vi "Auto Dispose.vi"(8 "error in (no error)":errorcluster, 11 "Progress Bar":refnum<data-value>) -> (0 "error out":errorcluster, 3 "Progress Bar":refnum<data-value>)   [LabVIEW 2016, in "Progress Bar.lvclass"]
doc: "If the reference was auto generated, then this VI will dispose of it when the progress bar is complete\n\nCopyright: MGI\nAuthored by: Derek Trepanier"
uses:
  <userlib>/_MGI/User Interface/Progress Bar/Progress Bar.lvclass
  <userlib>/_MGI/User Interface/Progress Bar/Progress Bar.lvclass/Progress Bar.ctl
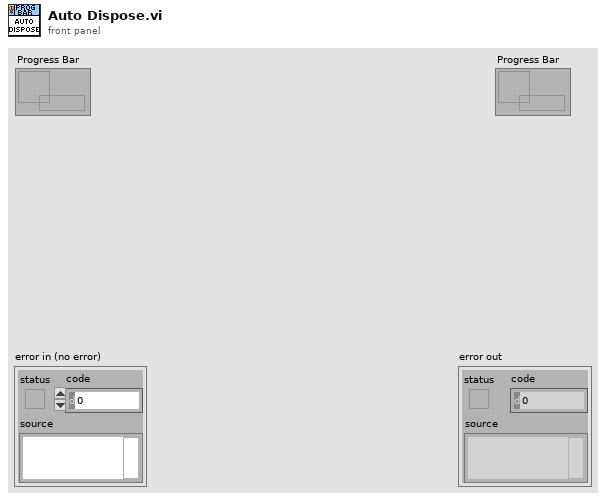
[diagram p1: front panel]
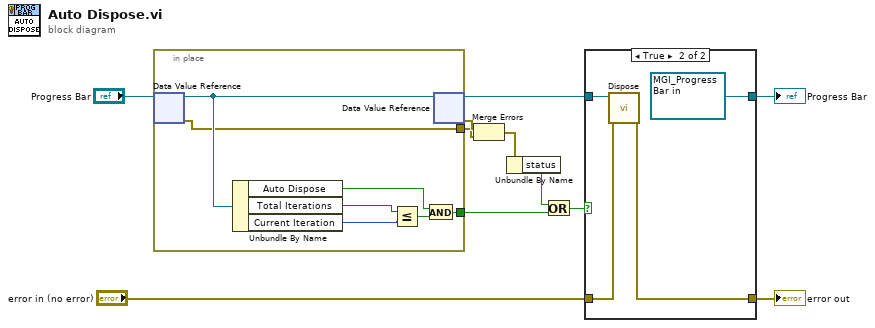
[diagram p0: block diagram]
diagram:
  n1 = in-place {
    in-place-border: [w14] -> w6
    in-place-border: [w13] -> w1
    n2 = in-place-dvr #1("Progress Bar") -> (w18:refnum<class "Progress Bar.lvclass">, w13:errorcluster)
    n3 = Unbundle By Name(w18) -> ("Auto Dispose"=w15:bool, "Total Iterations"=w17:i32, "Current Iteration"=w12:i32)
    n4 = Less Or Equal?(x=w17, y=w12) -> (x <= y?=w16:bool)
    n5 = And(x=w15, y=w16) -> (x .and. y?=w14:bool)
    n6 = in-place-dvr #1(w18) -> (w7:refnum<data-value>, w2:errorcluster)
  }
  n7 = Merge Errors(w2, w1) -> (w4:errorcluster)
  n8 = Unbundle By Name(w4) -> ("status"=w3:bool)
  n9 = Or(x=w3, y=w6) -> (x .or. y?=w5:bool)
  n10 = case shown="True" w5 {
    tunnel: [w20 refnum<data-value> refnum ("Progress Bar 2")] -> w11
    tunnel: w7 -> [w20 w23]
    tunnel: "error in (no error)" -> [w19 w22]
    tunnel: [w19 w21] -> w9
    frame False {
    }
    frame True {
      n11 = call <userlib>:"Dispose.vi"("error in (no error)"=w22, "Data Value Reference in"=w23) -> ("error out"=w21:errorcluster)  [unwired: 9 in]
    }
  }
  "error out" <- w9
  "Progress Bar" <- w11
